vi "VS Errors_Report Startup to Process.vi"(8 "Error":errorcluster, 11 "This VI":refnum<vi>) -> (0 "error out":errorcluster)   [LabVIEW 2021, in "CANOpen Addon Engine.lvlib"]
uses:
  CANOpen Addon Engine.lvlib
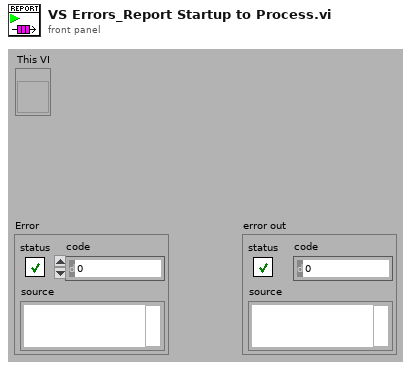
[diagram p1: front panel]
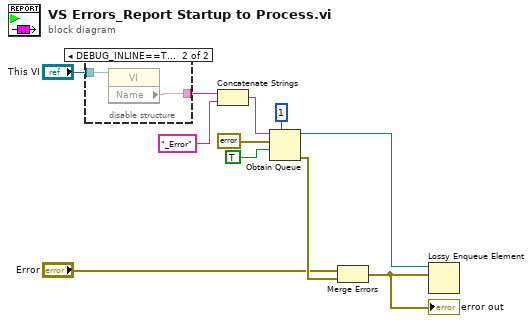
[diagram p0: block diagram]
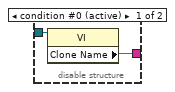
[diagram p2: hidden frame]
diagram:
  n1 = disable-structure shown="DEBUG_INLINE==TRUE" {
    disable-tunnel: "This VI" -> [w13 w15]
    disable-tunnel: [w12 w14] -> w9
    frame condition #0 (active) {
      n2 = property class="VI"(reference=w13) -> ("Clone Name"=w12:string)  [unwired: 1 in, 2 out]
    }
    frame condition #1 {
      n3 = property class="VI"(reference=w15) -> ("Name"=w14:string)  [unwired: 1 in, 2 out]
    }
  }
  n4 = Concatenate Strings(w9, "_Error" ("string")) -> (w7:string)
  n5 = Obtain Queue(max queue size (-1, unlimited)=1, name (unnamed)=w7, element data type=errorcluster {"status"=FALSE, "code"=0, "source"=""} ("error out"), create if not found? (T)=TRUE) -> (queue out=w10:refnum<queue>, error out=w3:errorcluster)  [unwired: 1 in, 1 out]
  n6 = Merge Errors("Error", w3) -> (w1:errorcluster)
  "error out" <- w1
  n7 = Lossy Enqueue Element(queue=w10, element=w1) -> ()  [unwired: 1 in, 4 out]
